vi "Stream No Loop.vi"() -> ()   [LabVIEW 2020]
panel:
  out "SampleRate (Hz)":dbl format="%.3f"
  out "NumAddresses":i32
  in  "STREAM_RESOLUTION_INDEX":i32
  in  "STREAM_SETTLING_US":i32
  in  "AIN_ALL_RANGE":dbl=10.0 format="%.3f"
  in  "NumScans":i32=2000
  out "ConnectionType Out":i32
  out "DeviceType Out":i32
  in  "Identifier":string="LJM_idANY"
  in  "ConnectionType":string="LJM_ctANY"
  in  "DeviceType":string="LJM_dtANY"
  out "Data":dbl[][](array[numeric]) format="%.3f"
  out "Waveform Graph":dbl[][](graph)
  in  "Scan List":string[](array[string])=["AIN0", "AIN1", "AIN2", "AIN3"]
  in  "Scan Rate (Hz)":dbl=1000.0 format="%.3f"
  out "Error Message":string
  # "To remove an element, right-click\non it, select Data Operations =>\nRemove Element.\n\nTo empty an array, right-click\nnear the edge, select Data\nOperations => Empty Array.\n\nOther useful operations:  From the\nOperate menu are \"Make Current\nValues Default\" and \"Reinitialize\nTo Default\"."
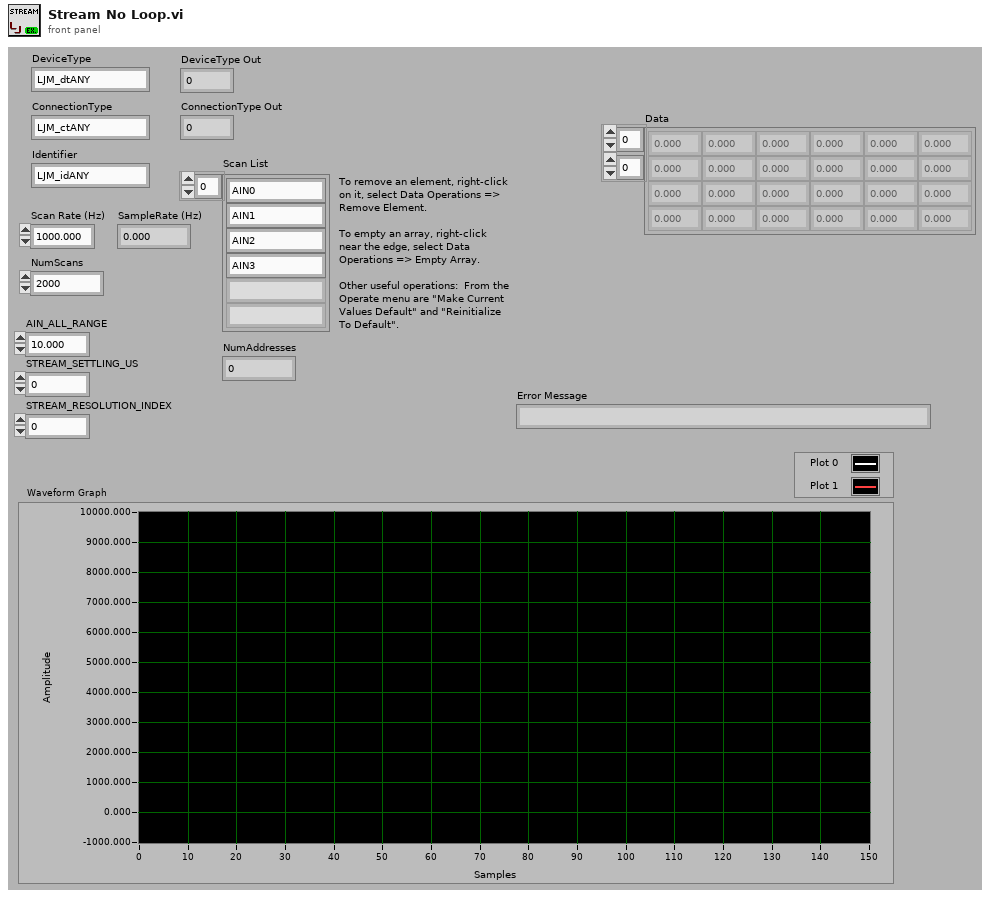
[diagram p1: front panel]
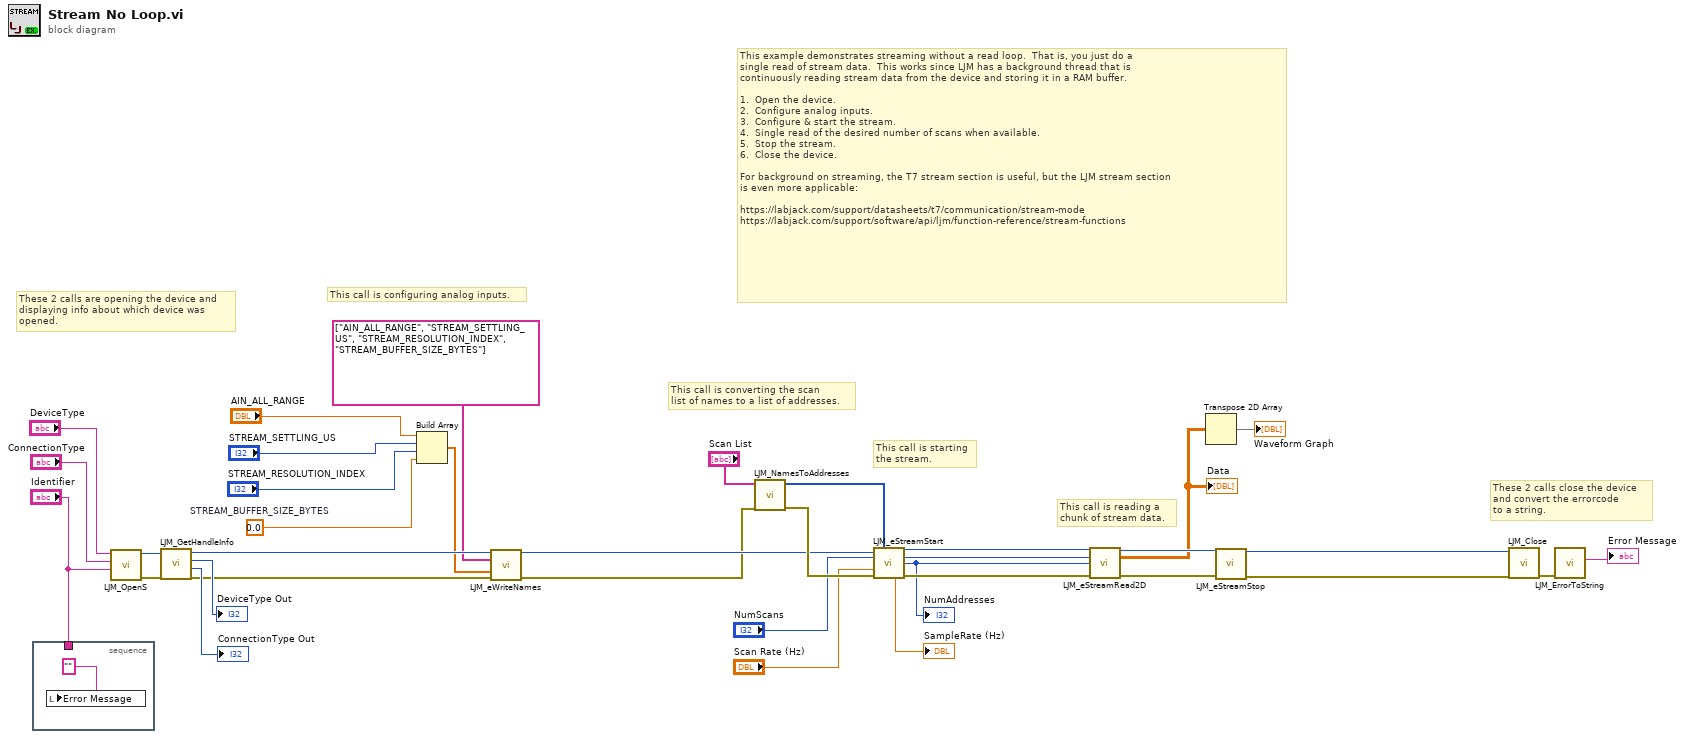
[diagram p0: block diagram]
diagram:
  w5 = 0.0  # STREAM_BUFFER_SIZE_BYTES
  # "This call is reading a\nchunk of stream data."
  # "This example demonstrates streaming without a read loop.  That is, you just do a\nsingle read of stream data.  This works since LJM has a background thread that is\ncontinuously reading stream data from the device and storing it in a RAM buffer.\n\n1.  Open the device.\n2.  Configure analog inputs.\n3.  Configure & start the stream.\n4.  Single read of the desired number of scans when available.\n5.  Stop the stream.\n6.  Close the device.\n\nFor background on streaming, the T7 stream section is useful, but the LJM stream section\nis even more applicable:\n\nhttps://labjack.com/support/datasheets/t7/communication/stream-mode\nhttps://labjack.com/support/software/api/ljm/function-reference/stream-functions"
  # "These 2 calls close the device\nand convert the errorcode\nto a string."
  # "This call is starting\nthe stream."
  # "This call is converting the scan\nlist of names to a list of addresses."
  # "This call is configuring analog inputs."
  # "These 2 calls are opening the device and\ndisplaying info about which device was\nopened."
  n1 = stacked-sequence {
    tunnel: "Identifier" -> [_]
    frame #0 {
      n2 = local write "Error Message"("" ("Error Message")) -> ()
    }
  }
  n3 = call "LJM_OpenS.vi"("Identifier"="Identifier", "ConnectionType"="ConnectionType", "DeviceType"="DeviceType") -> ("error out"=w27:errorcluster, "Handle"=w24:i32)  [unwired: 7 in]
  n4 = call "LJM_GetHandleInfo.vi"("error in"=w27, "Handle In"=w24) -> ("error out"=w19:errorcluster, "ConnectionType"=→"ConnectionType Out":i32, "DeviceType"=→"DeviceType Out":i32, "Handle Out"=w18:i32)  [unwired: 2 in, 4 out]
  n5 = Build Array("AIN_ALL_RANGE", "STREAM_SETTLING_US", "STREAM_RESOLUTION_INDEX", w5) -> (w13:dbl[])
  n6 = call "LJM_eWriteNames.vi"("Handle In"=w18, "aNames"=string[] ["AIN_ALL_RANGE", "STREAM_SETTLING_US", "STREAM_RESOLUTION_INDEX", "STREAM_BUFFER_SIZE_BYTES"], "aValuesIn"=w13, "error in"=w19) -> ("Handle Out"=w17:i32, "error out"=w16:errorcluster)  [unwired: 9 in, 1 out]
  n7 = call "LJM_NamesToAddresses.vi"("error in"=w16, "aNames"="Scan List") -> ("error out"=w20:errorcluster, "aAddresses"=w10:i32[])  [unwired: 7 in, 1 out]
  n8 = call "LJM_eStreamStart.vi"("Handle In"=w17, "aScanList"=w10, "ScansPerRead"="NumScans", "ScanRate"="Scan Rate (Hz)", "error in"=w20) -> ("Handle Out"=w34:i32, "ScansPerRead Out"=w6:i32, "NumReadAddresses"=w8:i32, "Actual SampleRate"=→"SampleRate (Hz)":dbl, "error out"=w35:errorcluster)  [unwired: 5 in, 1 out]
  "NumAddresses" <- w8
  n9 = call "LJM_eStreamRead2D.vi"("Handle In"=w34, "ScansPerRead"=w6, "NumAddresses"=w8, "error in"=w35) -> ("Handle Out"=w32:i32, "aData Out"=w1:dbl[][], "error out"=w33:errorcluster)  [unwired: 7 in, 2 out]
  "Data" <- w1
  n10 = Transpose 2D Array(2D array=w1) -> (transposed array=→"Waveform Graph":dbl[][])
  n11 = call "LJM_eStreamStop.vi"("Handle In"=w32, "error in"=w33) -> ("Handle Out"=w30:i32, "error out"=w31:errorcluster)  [unwired: 12 in]
  n12 = call "LJM_Close.vi"("error in"=w31, "Handle"=w30) -> ("error out"=w29:errorcluster)  [unwired: 9 in]
  n13 = call "LJM_ErrorToString.vi"("error in"=w29) -> ("String"=→"Error Message":string)  [unwired: 10 in]
